vi "csvBitWrite.vi"(5 "data buffer":string, 7 "valid data in buffer":i32, 8 "error in (no error)":errorcluster, 9 "CSV Formatted String":string, 11 "Byte Stream File in":refnum<file>) -> (0 "error out":errorcluster, 1 "Valid Data Buf OUT":i32, 2 "Data buffer OUT":string, 3 "Byte Stream File out":refnum<file>)   [LabVIEW 2019]
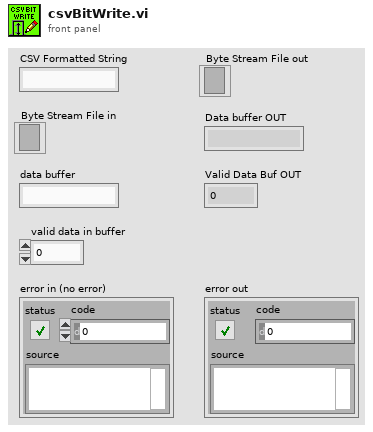
[diagram p1: front panel]
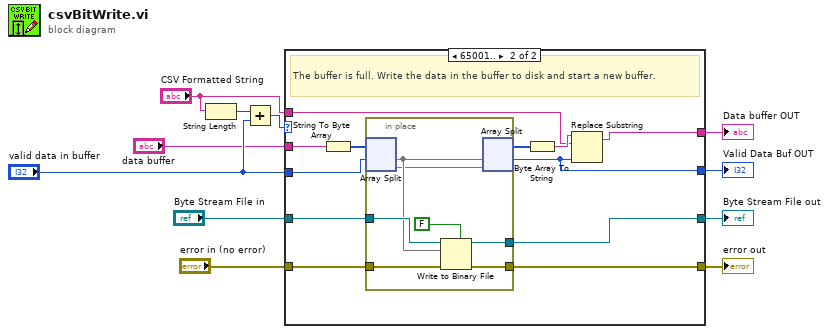
[diagram p0: block diagram]
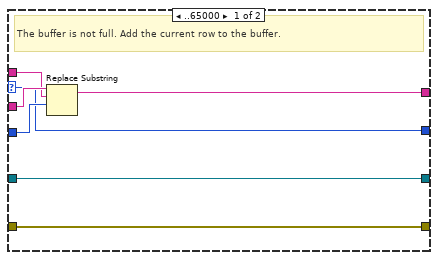
[diagram p2: hidden frame]
diagram:
  n1 = String Length(string="CSV Formatted String") -> (length=w6:i32)
  n2 = Add(x=w6, y="valid data in buffer") -> (x+y=w2:i32)
  n3 = case shown="65001.." w2 {
    selector: w2 -> [w12 _]
    tunnel: "error in (no error)" -> [w14 w28]
    tunnel: "CSV Formatted String" -> [w16 w21]
    tunnel: "data buffer" -> [w18 w26]
    tunnel: "valid data in buffer" -> [w17 w20]
    tunnel: [w15 w22] -> w7
    tunnel: [w14 w27] -> w11
    tunnel: [w13 w29] -> w8
    tunnel: "Byte Stream File in" -> [w13 w30]
    tunnel: [w12 w19] -> w10
    frame ..65000 {
      # "The buffer is not full. Add the current row to the buffer."
      n4 = Replace Substring(3:w17, 4:w16, 5:w18) -> (1:w15:string)  [unwired: 1 in, 1 out]
    }
    frame 65001.. {
      # "The buffer is full. Write the data in the buffer to disk and start a new buffer."
      n5 = String To Byte Array(string=w26) -> (unsigned byte array=w25:u8[])
      n6 = in-place {
        in-place-border: w30 -> [w37]
        in-place-border: [w36] -> w29
        in-place-border: w28 -> [w35]
        in-place-border: [w34] -> w27
        n7 = in-place-split #1(w25, w20) -> (w33:u8[], w32:u8[])
        n8 = Write to Binary File(file (use dialog)=w37, data=w33, error in=w35, 5:FALSE ("prepend array size")) -> (refnum out=w36:refnum<file>, error out=w34:errorcluster)  [unwired: 2 in, 1 out]
        n9 = in-place-split #1(w33, w32) -> (w24:u8[], w19:i32)
      }
      n10 = Byte Array To String(unsigned byte array=w24) -> (string=w23:string)
      n11 = Replace Substring(2:w19, 4:w21, 5:w23) -> (1:w22:string)  [unwired: 1 in, 1 out]
    }
  }
  "error out" <- w11
  "Valid Data Buf OUT" <- w10
  "Byte Stream File out" <- w8
  "Data buffer OUT" <- w7
